vi "VI Stoermeldungen.vi"() -> ()   [LabVIEW 2020, in "Stoerungen.lvlib"]
uses:
  Stoerungen/Stoerungen.lvlib
  Stoerungen/Stoermelde Tabelle.ctl
  Visualisierungs Elemente/Button.ctl
  Stoerungen/FGV Stoermeldungen Aktion.ctl
  Stoerungen/FGV Stoerungsdatei Aktionen.ctl
  Stoerungen/FGV Stoerung aufnehmen Aktion.ctl
  Allgemein/allgemeine Sub-VIs.lvlib
panel:
  in  "quittieren":T1
  out "Tabelle":T2
  # "Störmeldungen"
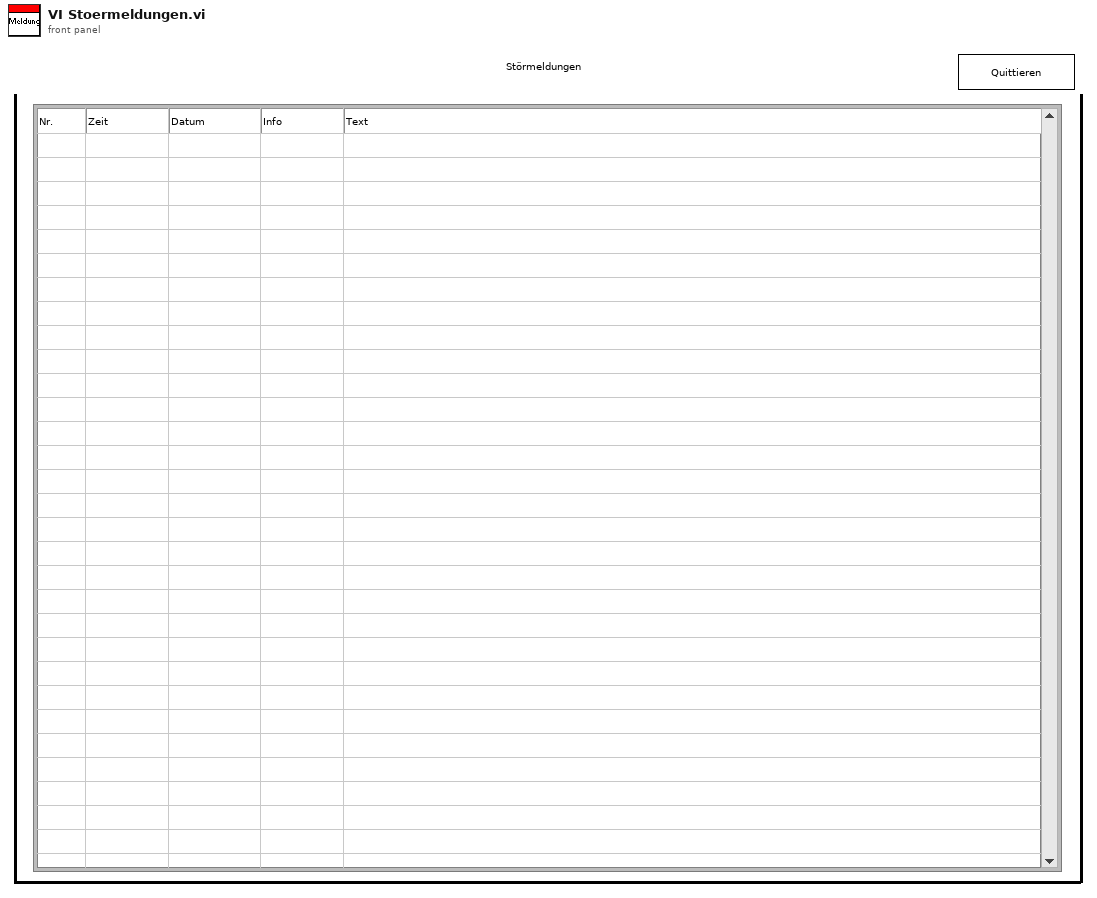
[diagram p1: front panel]
types:
  T1 = typedef "Button.ctl" = bool
  T2 = typedef "Stoerungen.lvlib/Stoermelde Tabelle.ctl" = string[][]
  T3 = typedef "Stoerungen.lvlib/FGV Stoerungsdatei Aktionen.ctl" = enum16{"lesen", "laden", "Neue Werte"}
  T4 = typedef "Stoerungen.lvlib/FGV Stoermeldungen Aktion.ctl" = enum16{"Initialisieren", "kommend", "gehend", "lesen", "Queue leeren", "Queue freigeben", "in Datei loggen", "Änderung zurücksetzen"}
  T5 = typedef "Stoerungen.lvlib/Stoermeldung.ctl" = cluster{"Zeitstempel":timestamp, "Nummer":i32, "Kommend":bool}
  T6 = typedef "Stoerungen.lvlib/FGV Stoerung aufnehmen Aktion.ctl" = enum16{"Initialisieren", "Schreiben", "Lesen", "Quittieren", "quit. löschen"}
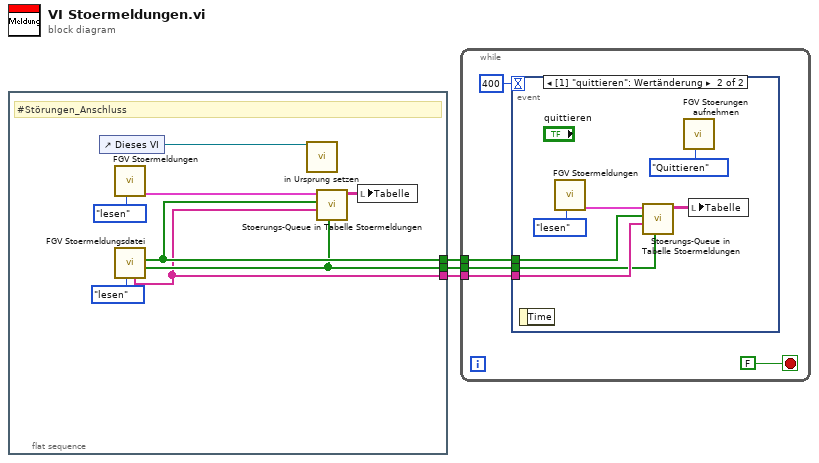
[diagram p0: block diagram]
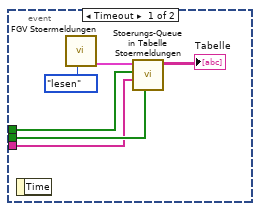
[diagram p2: hidden frame]
diagram:
  n1 = flat-sequence {
    tunnel: [w4] -> w3
    tunnel: [w9] -> w2
    tunnel: [w7] -> w1
    frame #0 {
      # "#Störungen_Anschluss"
      n2 = control-ref of="Dieses VI"() -> (w5:refnum<vi>)
      n3 = call "FGV Stoermeldungen.vi"("Aktion"=FGV_Stoermeldungen_Aktion."lesen") -> ("Anzeige Array"=w6:T5[])  [unwired: 3 in, 7 out]
      n4 = call "FGV Stoermeldungsdatei.vi"("Aktionen"=FGV_Stoerungsdatei_Aktionen."lesen") -> ("abschaltend"=w7:bool[], "quittieren?"=w9:bool[], "Text"=w4:string[])  [unwired: 2 in, 6 out]
      n5 = call "in Ursprung setzen.vi"("VI Referenz"=w5) -> ()  [unwired: 10 in, 1 out]
      n6 = call "Stoerungs-Queue in Tabelle Stoermeldungen.vi"("Abschalten aus Datei"=w7, "Störmeldetexte aus Datei"=w4, "Quittieren aus Datei"=w9, "Queue-Inhalt\n(FGV Störmeldungen)"=w6) -> ("Tabelle Störmeldungen"=w10:string[][])  [unwired: 1 in, 6 out]
      n7 = local write "Tabelle"(w10) -> ()
    }
  }
  n8 = while {
    tunnel: w3 -> [w15]
    tunnel: w2 -> [w14]
    tunnel: w1 -> [w13]
    stop <- FALSE stop-if-true
    n9 = event shown="[1] \"quittieren\": Wertänderung" {
      selector: _ -> [_ _]
      dyn-events: _ -> [_ _]
      timeout: 400 -> [_ _]
      tunnel: w15 -> [w17 w26]
      tunnel: w14 -> [w19 w27]
      tunnel: w13 -> [w18 w24]
      event Timeout {
        n10 = event-data() -> ()  [unwired: 2 out]
        n11 = call "FGV Stoermeldungen.vi"("Aktion"=FGV_Stoermeldungen_Aktion."lesen") -> ("Anzeige Array"=w20:T5[])  [unwired: 3 in, 7 out]
        n12 = call "Stoerungs-Queue in Tabelle Stoermeldungen.vi"("Abschalten aus Datei"=w18, "Störmeldetexte aus Datei"=w17, "Quittieren aus Datei"=w19, "Queue-Inhalt\n(FGV Störmeldungen)"=w20) -> ("Tabelle Störmeldungen"=→"Tabelle":string[][])  [unwired: 1 in, 6 out]
      }
      event Value Change {
        n13 = event-data() -> ()  [unwired: 2 out]
        n14 = call "FGV Stoermeldungen.vi"("Aktion"=FGV_Stoermeldungen_Aktion."lesen") -> ("Anzeige Array"=w23:T5[])  [unwired: 3 in, 7 out]
        n15 = call "Stoerungs-Queue in Tabelle Stoermeldungen.vi"("Abschalten aus Datei"=w24, "Störmeldetexte aus Datei"=w26, "Quittieren aus Datei"=w27, "Queue-Inhalt\n(FGV Störmeldungen)"=w23) -> ("Tabelle Störmeldungen"=w29:string[][])  [unwired: 1 in, 6 out]
        n16 = call "FGV Stoerungen aufnehmen.vi"("FGV Störung aufnehmen Aktion"=FGV_Stoerung_aufnehmen_Aktion."Quittieren") -> ()  [unwired: 7 in, 4 out]
        n17 = local write "Tabelle"(w29) -> ()
      }
    }
  }
